vi "18.2.3 Matching-Inspection.vi"() -> ()   [LabVIEW 2017]
doc: "This example illustrates the use of the horizontal clamp tool. You can draw a region of inspection that contains at least two edges in the image. The VI measures the distance between the first and last edges."
uses:
  <vilib>/vision/NI_Vision_Development_Module.lvlib
panel:
  in  "stop":bool
  in  "Delay(s)":dbl(slide)=1.0285714285714285 scale=0.0..3.0
  out "Pass？":bool
  out "Match Flag":bool[](array[boolean])
  out "Match Score":i32[](array[numeric])
  out "UUT":T1(plugin-control)
  out "TMP":T1(plugin-control)
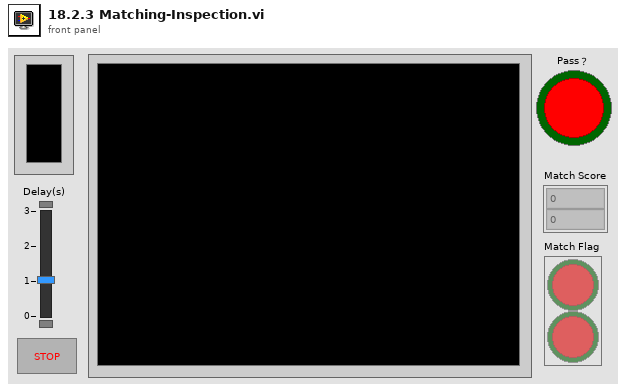
[diagram p1: front panel]
types:
  T1 = typedef "IMAQ Image.ctl" = refnum<image>
  T2 = typedef "ROI Descriptor" = cluster{"Global Rectangle":i32[], "Contours":cluster{"ID":enum32{"External", "Internal"}, "Type":u32, "Coordinates":i32[]}[]}
  T3 = typedef "Image Type" = u32
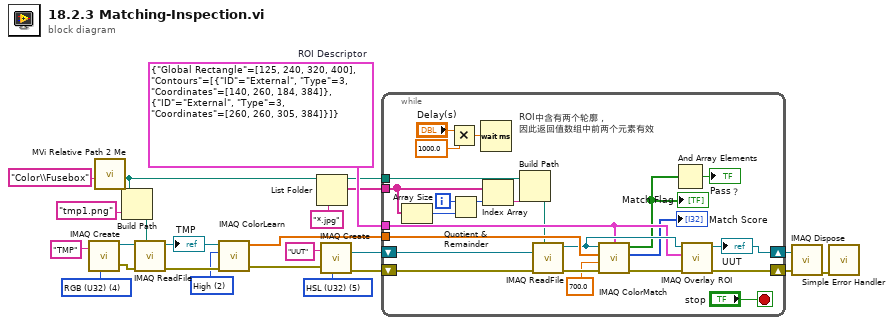
[diagram p0: block diagram]
diagram:
  w5 = T2 {"Global Rectangle"=[125, 240, 320, 400], "Contours"=[{"ID"=enum."External", "Type"=3, "Coordinates"=[140, 260, 184, 384]}, {"ID"=enum."External", "Type"=3, "Coordinates"=[260, 260, 305, 384]}]}  # ROI Descriptor
  w12 = u32 2 items=["Low", "Medium", "High"] ("Color Sensitivity")
  w19 = T3 5 items=["Grayscale (U8)", "Grayscale (I16)", "Grayscale (SGL)", "Complex (CSG)", "RGB (U32)", "HSL (U32)", "RGB (U64)", "Grayscale (U16)"] ("Image Type")
  w21 = T3 4 items=["Grayscale (U8)", "Grayscale (I16)", "Grayscale (SGL)", "Complex (CSG)", "RGB (U32)", "HSL (U32)", "RGB (U64)", "Grayscale (U16)"] ("Image Type")
  n1 = call "IMAQ Create"("Image Name"="TMP", "Image Type"=w21) -> ("New Image"=w20:T1, "error out"=w11:errorcluster)  [unwired: 3 in]
  n2 = call "MVi Relative Path 2 Me.vi"("Relative Path"="Color\\Fusebox" ("name or relative path")) -> ("Appended Dir"=w4:path)  [unwired: 5 in, 1 out]
  n3 = Build Path(base path=w4, name or relative path="tmp1.png") -> (appended path=w9:path)
  n4 = call "IMAQ ReadFile"("File Path"=w9, "error in (no error)"=w11, "Image"=w20) -> ("error out"=w13:errorcluster, "Image Out"=w8:T1)  [unwired: 4 in, 3 out]
  "TMP" <- w8
  n5 = call "IMAQ ColorLearn"("Image"=w8, "Color Sensitivity"=w12, "error in (no error)"=w13) -> ("Color Spectrum"=w14:dbl[], "error out"=w15:errorcluster)  [unwired: 5 in]
  n6 = List Folder(path=w4, pattern="*.jpg") -> (path out=w2:path, filenames=w1:string[])  [unwired: 2 in, 2 out]
  n7 = call "IMAQ Create"("Image Name"="UUT", "Image Type"=w19, "error in (no error)"=w15) -> ("New Image"=w17:T1, "error out"=w16:errorcluster)  [unwired: 2 in]
  n8 = while {
    tunnel: w14 -> [w45]
    tunnel: w5 -> [w39]
    shift-right: [w40] -> w6
    shift-left: w17 -> [w48]
    shift-right: [w42] -> w7
    shift-left: w16 -> [w47]
    tunnel: w2 -> [w35]
    tunnel: w1 -> [w28]
    i -> [w30]
    stop <- "stop" stop-if-true
    # "ROI中含有两个轮廓，\n因此返回值数组中前两个元素有效"
    n9 = Array Size(array=w28) -> (size(s)=w29:i32)
    n10 = Multiply(x="Delay(s)", y=1000.0) -> (x*y=w31:dbl)
    n11 = Quotient & Remainder(x=w30, y=w29) -> (x-y*floor(x/y)=w25:i32)  [unwired: 1 out]
    n12 = Wait (ms)(milliseconds to wait=w31) -> ()  [unwired: 1 out]
    n13 = Index Array(array=w28, index=w25) -> (element=w27:string)
    n14 = Build Path(base path=w35, name or relative path=w27) -> (appended path=w34:path)
    n15 = call "IMAQ ReadFile"("File Path"=w34, "error in (no error)"=w47, "Image"=w48) -> ("error out"=w46:errorcluster, "Image Out"=w41:T1)  [unwired: 4 in, 3 out]
    n16 = call "IMAQ ColorMatch"("ROI Descriptor"=w39, "Image"=w41, "Color Spectrum"=w45, "Minimum Match Score"=700.0, "error in (no error)"=w46) -> ("Match Flag"=w37:bool[], "Match Score"=→"Match Score":i32[], "error out"=w43:errorcluster)  [unwired: 1 in, 1 out]
    "Match Flag" <- w37
    n17 = And Array Elements(Boolean array=w37) -> (logical AND=→"Pass？":bool)
    n18 = call "IMAQ Overlay ROI"("error in (no error)"=w43, "ROI Descriptor"=w39, "Image"=w41) -> ("error out"=w42:errorcluster, "Image Out"=w40:T1)  [unwired: 7 in]
    "UUT" <- w40
  }
  n19 = call "IMAQ Dispose"("Image"=w6, "error in (no error)"=w7) -> ("error out"=w24:errorcluster)  [unwired: 4 in]
  n20 = call <vilib>:"Simple Error Handler.vi"("error in (no error)"=w24) -> ()  [unwired: 4 in, 5 out]
